vi "set current and voltage.vi"(0 "Voltage":dbl format="%.2f", 1 "VISA Resource Name":refnum<visa-resource-name>, 2 "Current":dbl format="%.2f", 3 "OVP":dbl format="%.2f", 4 "Power":bool, 5 "OCP":dbl format="%.2f") -> (6 "Voltage":string, 7 "Current":string)   [LabVIEW 2009]
doc: "This VI form sets all the set points for the current memory location.\nDESCRIPTION:\nThis VI configures the power supplies to generate a DV voltage at the output.\n\nINSTRUCTIONS:\n1. Enter the resource name.\n2. Enter voltage level, current limit, OVP limit and OCP limit.\n3. Set output enabled switch to ON if you want the generated voltage to appear at the instrument's output.\n4. Run the VI."
panel:
  out "error out":errorcluster
  in  "error in (no error)":errorcluster
  # "MAGNA-POWER"
  # "Electronics"
  # "ON"
  # "OFF"
  # "Instrument Settings"
  # "Output Values"
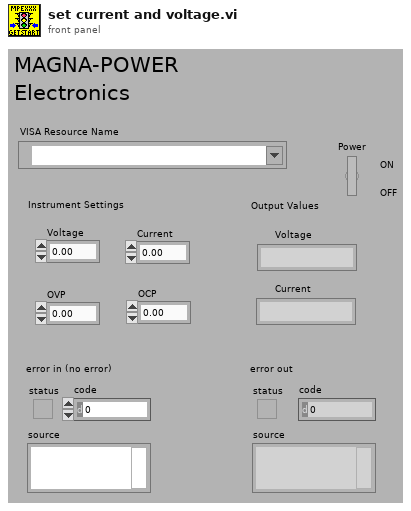
[diagram p1: front panel]
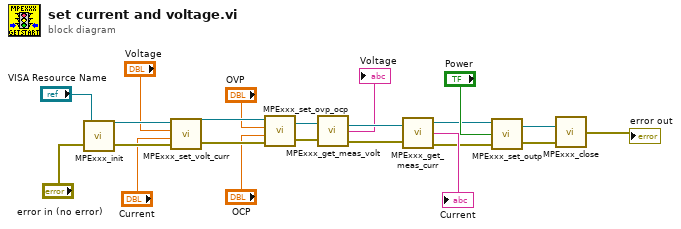
[diagram p0: block diagram]
diagram:
  n1 = call "MPExxx_init.vi"("error in (no error)"="error in (no error)", "VISA session"="VISA Resource Name") -> ("error out"=w21:errorcluster, "dup VISA session"=w14:refnum<visa-resource-name>)
  n2 = call "MPExxx_set_volt_curr.vi"("error in (no error)"=w21, "Set Current"="Current", "Set Voltage"="Voltage", "VISA session"=w14) -> ("error out"=w20:errorcluster, "dup VISA session"=w15:refnum<visa-resource-name>)
  n3 = call "MPExxx_set_ovp_ocp.vi"("error in (no error)"=w20, "Set OCP"="OCP", "Set OVP"="OVP", "VISA session"=w15) -> ("error out"=w19:errorcluster, "dup VISA session"=w16:refnum<visa-resource-name>)
  n4 = call "MPExxx_get_meas_volt.vi"("VISA session"=w16, "error in (no error)"=w19) -> ("dup VISA session"=w17:refnum<visa-resource-name>, "Output Voltage"=→"Voltage":string, "error out"=w18:errorcluster)
  n5 = call "MPExxx_get_meas_curr.vi"("VISA session"=w17, "error in (no error)"=w18) -> ("dup VISA session"=w4:refnum<visa-resource-name>, "Output Current"=→"Current":string, "error out"=w3:errorcluster)
  n6 = call "MPExxx_set_outp.vi"("error in (no error)"=w3, "Output Control"="Power", "VISA session"=w4) -> ("error out"=w2:errorcluster, "dup VISA session"=w1:refnum<visa-resource-name>)
  n7 = call "MPExxx_close.vi"("error in (no error)"=w2, "VISA session"=w1) -> ("error out"=→"error out":errorcluster)
